vi "FaradayCupStatusChange.vi"(8 "error in (no error)":errorcluster, 10 "ControlQueue":refnum<queue>, 11 "DAQmxTaskContainer in":refnum<class "DAQmxTaskContainer.lvclass">) -> (0 "error out":errorcluster, 3 "DAQmxTaskContainer out":refnum<class "DAQmxTaskContainer.lvclass">)   [LabVIEW 2015, in "DAQmxTaksContainer_General.lvclass"]
uses:
  DAQmxTaksContainer_General.lvclass
  DAQmxTask.lvclass
  dependecies/ControlsVIs/Clusters-def/ProtypeCommand-DAQmxReply.ctl
  dependecies/ControlsVIs/Clusters-def/SERVER-Commands.ctl
  Control/Control-Server/Control-Server.lvclass
  dependecies/ControlsVIs/Clusters-def/Standard Command.ctl
  Message/Message.lvclass
  dependecies/ControlsVIs/Clusters-def/Message types.ctl
  GeneralFunctionality/GeneralFunctionality.lvclass
  DAQmxTaskContainer/DAQmxTaskContainer.lvclass
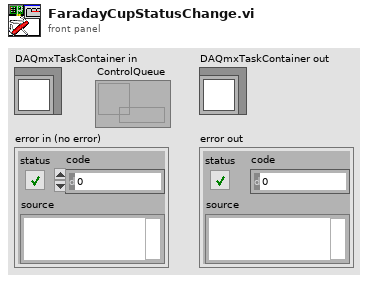
[diagram p1: front panel]
types:
  T1 = typedef "Message types.ctl" = string
  T2 = typedef "Standard Command.ctl" = cluster{"command":string, "data":variant}
  T3 = typedef "Control-Server.lvclass/SERVER-Commands.ctl" = string
  T4 = typedef "ProtypeCommand-DAQmxReply.ctl" = cluster{"On/Off":bool, "error out":errorcluster}
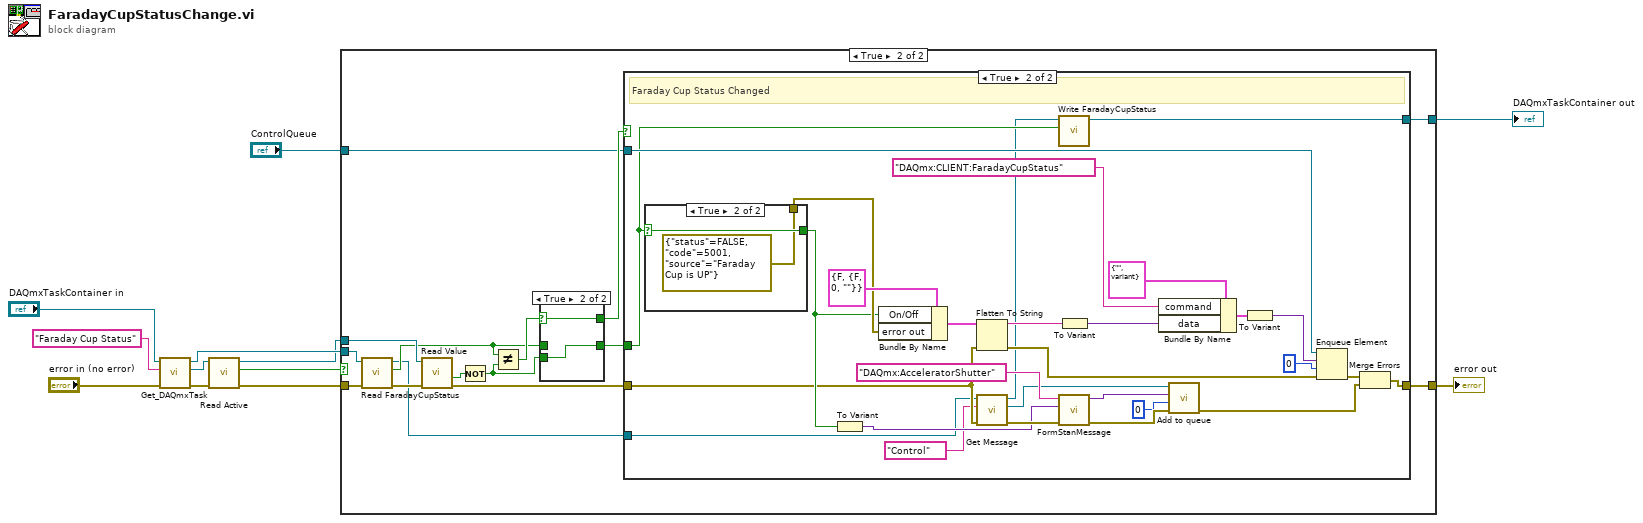
[diagram p0: block diagram]
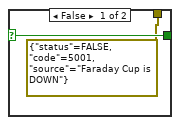
[diagram p4: hidden frame]
diagram:
  n1 = call "Get_DAQmxTask.vi"("error in (no error)"="error in (no error)", "Task name"="Faraday Cup Status", "DAQmxTaksContainer_General in"="DAQmxTaskContainer in") -> ("error out"=w5:errorcluster, "DAQmx Task"=w7:refnum<class "DAQmxTask.lvclass">, "DAQmxTaksContainer_General out"=w10:refnum<class "DAQmxTaskContainer.lvclass">)  [unwired: 6 in]
  n2 = call-dynamic "Read Active.vi"("error in (no error)"=w5, "DAQmxTask in"=w7) -> ("error out"=w8:errorcluster, "Active?"=w6:bool, "DAQmxTask out"=w9:refnum<class "DAQmxTask.lvclass">)  [unwired: 7 in]
  n3 = case shown="True" w6 {
    tunnel: w8 -> [w14 w18]
    tunnel: w9 -> [_ w29]
    tunnel: w10 -> [w13 w16]
    tunnel: [w14 w23] -> w12
    tunnel: [w13 w22] -> w11
    tunnel: "ControlQueue" -> [_ w21]
    frame False {
    }
    frame True {
      n4 = call "Read FaradayCupStatus.vi"("error in (no error)"=w18, "DAQmxTaksContainer_General in"=w16) -> ("error out"=w17:errorcluster, "FaradayCupStatus"=w19:bool, "DAQmxTaksContainer_General out"=w15:refnum<class "DAQmxTaskContainer.lvclass">)  [unwired: 7 in]
      n5 = call-dynamic "Read Value.vi"("error in (no error)"=w17, "DAQmxTask en entrée"=w29) -> ("error out"=w24:errorcluster, "Data"=w27:bool)  [unwired: 6 in, 2 out]
      n6 = Not(x=w27) -> (.not. x?=w20:bool)
      n7 = Not Equal?(x=w19, y=w20) -> (x != y?=w28:bool)
      n8 = case shown="True" w28 {
        selector: w28 -> [w65 w67]
        tunnel: [w66 w68] -> w25
        tunnel: w19 -> [w66 _]
        tunnel: w20 -> [_ w68]
        tunnel: [w65 w67] -> w26
        frame False {
        }
        frame True {
        }
      }
      n9 = case shown="True" w26 {
        tunnel: [w31 w33] -> w22
        tunnel: w25 -> [_ w34]
        tunnel: w15 -> [w31 w35]
        tunnel: w24 -> [w30 w38]
        tunnel: [w30 w48] -> w23
        tunnel: w21 -> [_ w47]
        frame False {
        }
        frame True {
          # "Faraday Cup Status Changed"
          n10 = case shown="True" w34 {
            selector: w34 -> [w62 w64]
            tunnel: [w62 w64] -> w39
            tunnel: [errorcluster {"status"=FALSE, "code"=5001, "source"="Faraday Cup is DOWN"} ("error out") errorcluster {"status"=FALSE, "code"=5001, "source"="Faraday Cup is UP"} ("error out")] -> w55
            frame False {
            }
            frame True {
            }
          }
          n11 = To Variant(anything=w39) -> (Variant=w41:variant)
          n12 = Bundle By Name(cluster=T4 {"On/Off"=FALSE, "error out"={"status"=FALSE, "code"=0, "source"=""}} ("output cluster"), "On/Off"=w39, "error out"=w55) -> (w59:T4)
          n13 = Flatten To String(anything=w59, error in (no error)=w38) -> (data string=w57:string, error out=w54:errorcluster)  [unwired: 2 in, 1 out]
          n14 = call "Get Message.vi"("error in (no error)"=w38, "Message type"=T1 "Control", "GeneralFunctionality en entrée"=w35) -> ("error out"=w46:errorcluster, "Message.lvclass"=w36:refnum<class "Message.lvclass">, "GeneralFunctionality en sortie"=w32:refnum<class "DAQmxTaskContainer.lvclass">)  [unwired: 6 in]
          n15 = call "Write FaradayCupStatus.vi"("FaradayCupStatus"=w34, "DAQmxTaksContainer_General in"=w32) -> ("DAQmxTaksContainer_General out"=w33:refnum<class "DAQmxTaskContainer.lvclass">)  [unwired: 8 in, 1 out]
          n16 = call "FormStanMessage.vi"("error in"=w46, "data"=w41, "Command"="DAQmx:AcceleratorShutter") -> ("error out"=w45:errorcluster, "message"=w44:variant)  [unwired: 7 in]
          n17 = To Variant(anything=w57) -> (Variant=w58:variant)
          n18 = Bundle By Name(cluster=T2 {"command"="", "data"=variant} ("input cluster"), "command"=T3 "DAQmx:CLIENT:FaradayCupStatus" ("Commands"), "data"=w58) -> (w53:T2)
          n19 = call "Add to queue.vi"("error in (no error)"=w45, "timeout in ms (-1)"=0, "Data"=w44, "Message in"=w36) -> ("error out"=w40:errorcluster)  [unwired: 6 in, 1 out]
          n20 = To Variant(anything=w53) -> (Variant=w52:variant)
          n21 = Enqueue Element(queue=w47, element=w52, timeout in ms (-1)=0 ("timeout en ms (-1)"), error in (no error)=w54) -> (error out=w49:errorcluster)  [unwired: 2 out]
          n22 = Merge Errors(w49, w40) -> (w48:errorcluster)
        }
      }
    }
  }
  "error out" <- w12
  "DAQmxTaskContainer out" <- w11
